vi "Mark Phonation Cutoff.vi"(7 "Error In":errorcluster, 8 "File Path":path, 10 "Pressure/Audio":dynamicdata(graph)) -> (0 "Error Out":errorcluster, 1 "File Path Indicator":path, 2 "Skip?":bool, 3 "Cutoff Pressures":dbl[](array[numeric]))   [LabVIEW 2018, in "AnalysisSupport.lvlib"]
uses:
  AnalysisSupport.lvlib
  <vilib>/Waveform/WDTOps.llb/WDT Get XY Value DBL.vi
panel:
  in  "Jump Button":bool
  in  "Show Audio":bool
  in  "Show EGG":bool
  in  "Undo Button":bool
  out "SPL":dbl
  in  "Help Button":bool
  in  "Add":bool
  out "Interruptions Marked":dbl
  out "Interruption Time":dbl
  in  "Done":bool
  out "Pressure":dbl
  out "EXIT":bool
  out "Enlarged":dynamicdata(graph)
  out "Pressure/Audio":dynamicdata(graph)
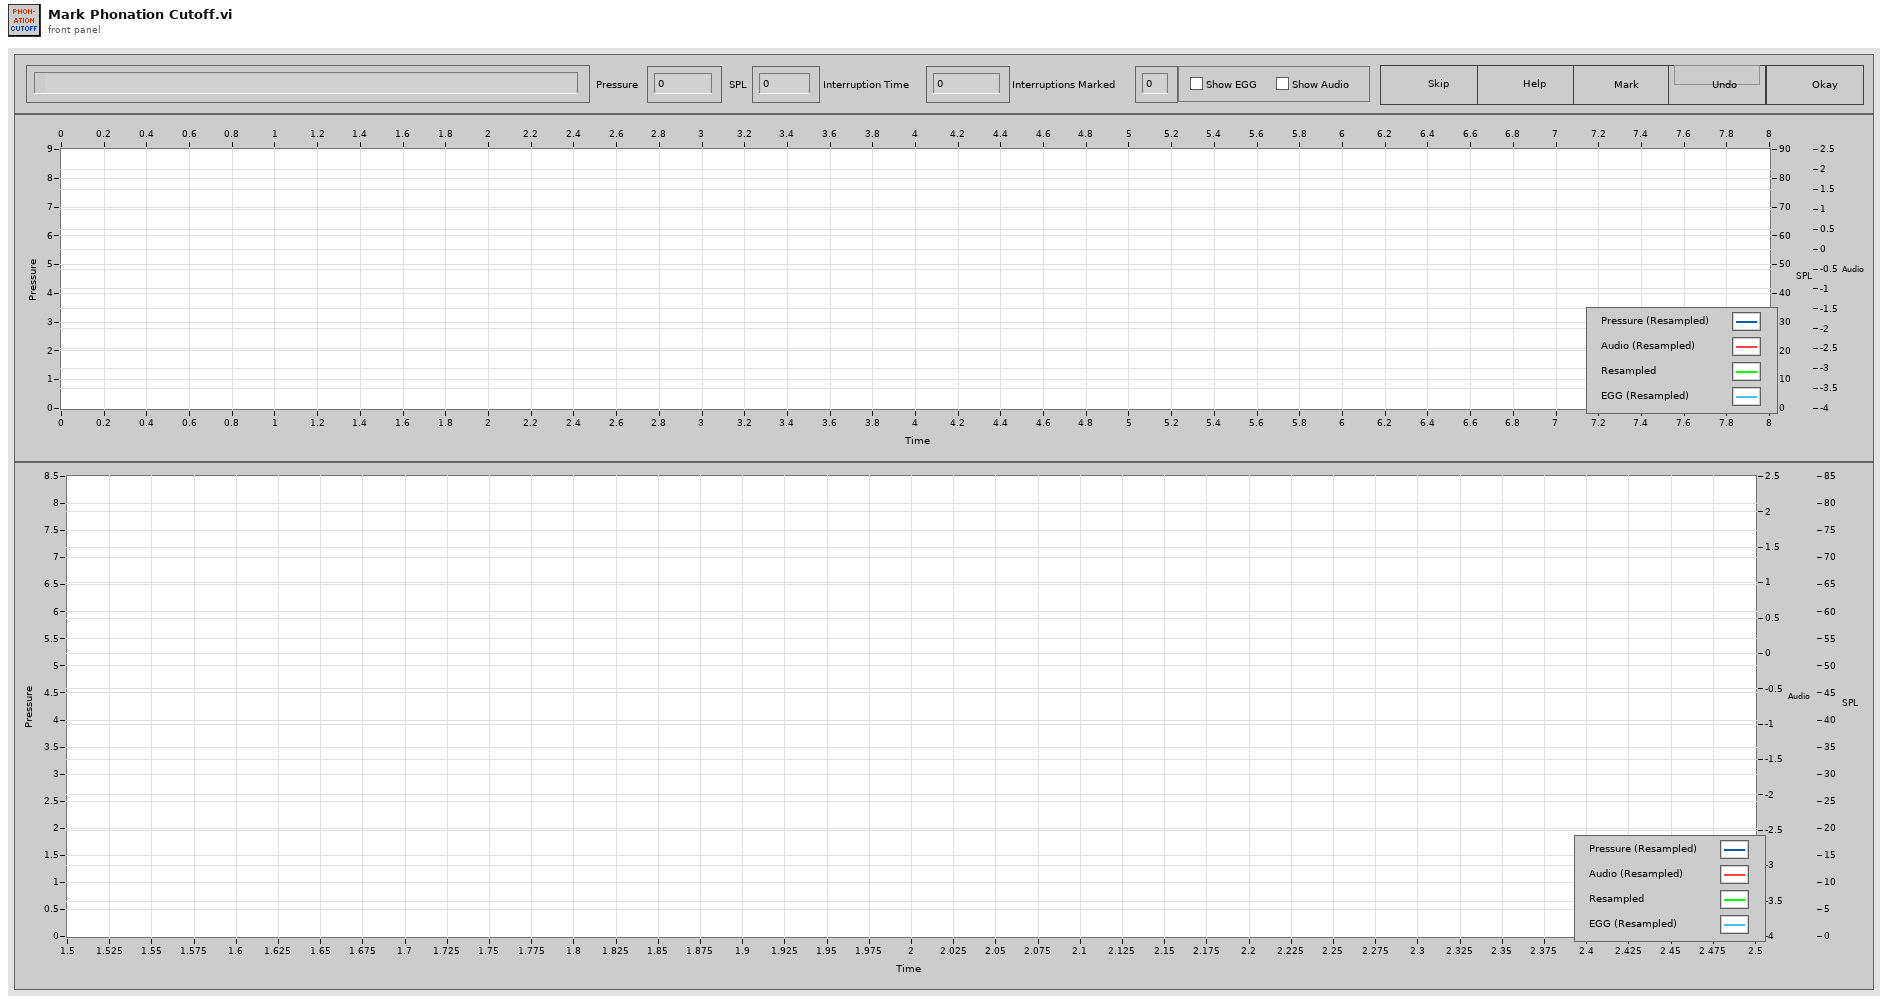
[diagram p1: front panel]
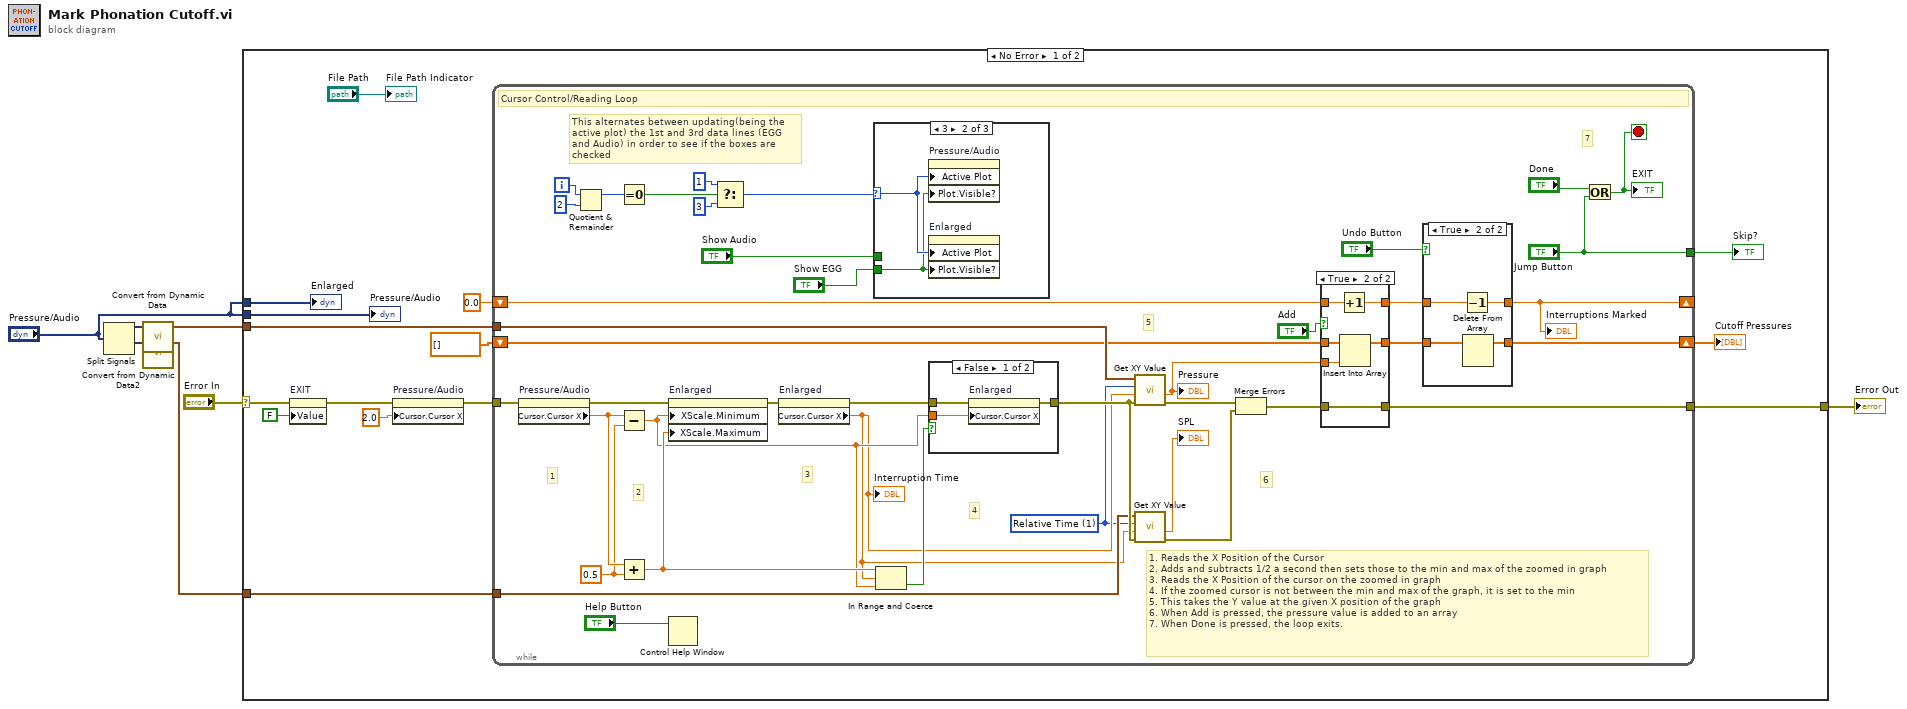
[diagram p0: block diagram]
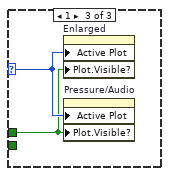
[diagram p3: hidden frame]
diagram:
  n1 = Split Signals("Pressure/Audio") -> (w4:dynamicdata, w2:dynamicdata)  [unwired: 4 in, 2 out]
  n2 = call "Convert from Dynamic Data"("Dynamic Data Type"=w4) -> ("Waveform"=w5:waveform(dbl))  [unwired: 3 in]
  n3 = call "Convert from Dynamic Data2"("Dynamic Data Type"=w2) -> ("Waveform"=w3:waveform(dbl))  [unwired: 3 in]
  n4 = case shown="No Error" "Error In" {
    selector: "Error In" -> [w11 w87]
    tunnel: [w21 w87] -> w7
    tunnel: "Pressure/Audio" -> [w16 _]
    tunnel: "Pressure/Audio" -> [w18 _]
    tunnel: w5 -> [w17 _]
    tunnel: w3 -> [w9 _]
    frame No Error {
      n5 = property on="EXIT" class="Bool (strict)"(error in=w11, "Value"=FALSE ("EXIT")) -> (error out=w10:errorcluster)  [unwired: 1 in, 1 out]
      n6 = property on="Pressure/Audio" class="WFGraph (strict)"(error in=w10, "Cursor.Cursor X"=2.0 ("Cursor.Cursor Position:Cursor X")) -> (error out=w19:errorcluster)  [unwired: 1 in, 1 out]
      n7 = while {
        tunnel: [w53] -> w21
        tunnel: w19 -> [w63]
        tunnel: w17 -> [w62]
        shift-right: [w38] -> _
        shift-left: 0.0 -> [w52]
        shift-right: [w36] -> w13
        shift-left: dbl[] [] ("Cutoff Pressures") -> [w50]
        tunnel: w9 -> [w42]
        tunnel: ["Jump Button"] -> w8
        i -> [w34]
        stop <- w25 stop-if-true
        w40 = u16 1 items=["Samples", "Relative Time"] ("Y position format")
        w59 = 0.5 ("y")
        # "This alternates between updating(being the active plot) the 1st and 3rd data lines (EGG and Audio) in order to see if the boxes are checked"
        # "6"
        # "5"
        # "7"
        # "4"
        # "3"
        # "2"
        # "1"
        # "1. Reads the X Position of the Cursor\n2. Adds and subtracts 1/2 a second then sets those to the min and max of the zoomed in graph\n3. Reads the X Position of the cursor on the zoomed in graph\n4. If the zoomed cursor is not between the min and max of the graph, it is set to the min\n5. This takes the Y value at the given X position of the graph\n6. When Add is pressed, the pressure value is added to an array\n7. When Done is pressed, the loop exits."
        # "Cursor Control/Reading Loop"
        n8 = property on="Pressure/Audio" class="WFGraph (strict)"(error in=w63) -> (error out=w57:errorcluster, "Cursor.Cursor X"=w60:dbl)  [unwired: 1 in, 1 out]
        n9 = Quotient & Remainder(x=w34, y=2) -> (x-y*floor(x/y)=w32:i32)  [unwired: 1 out]
        n10 = Equal To 0?(x=w32) -> (x = 0?=w31:bool)
        n11 = Subtract(x=w60, y=w59) -> (x-y=w54:dbl)
        n12 = Add(x=w60, y=w59) -> (x+y=w58:dbl)
        n13 = Control Help Window(1:"Help Button") -> ()  [unwired: 1 in]
        n14 = property on="Enlarged" class="WFGraph (strict)"(error in=w57, "XScale.Minimum"=w54, "XScale.Maximum"=w58) -> (error out=w56:errorcluster)  [unwired: 1 in, 1 out]
        n15 = Select(t=u32 1 ("Active Plot"), s=w31, f=u32 3 ("Active Plot")) -> (s? t:f=w28:u32)
        n16 = property on="Enlarged" class="WFGraph (strict)"(error in=w56) -> (error out=w55:errorcluster, "Cursor.Cursor X"=w41:dbl)  [unwired: 1 in, 1 out]
        "Interruption Time" <- w41
        n17 = case shown="3" w28 {
          selector: w28 -> [_ w65 w67]
          tunnel: "Show EGG" -> [_ w64 _]
          tunnel: "Show Audio" -> [_ _ w66]
          frame 0, Default {
          }
          frame 3 {
            n18 = property on="Pressure/Audio" class="WFGraph (strict)"("Active Plot"=w65, "Plot.Visible?"=w64) -> ()  [unwired: 2 in, 2 out]
            n19 = property on="Enlarged" class="WFGraph (strict)"("Active Plot"=w65, "Plot.Visible?"=w64) -> ()  [unwired: 2 in, 2 out]
          }
          frame 1 {
            n20 = property on="Enlarged" class="WFGraph (strict)"("Active Plot"=w67, "Plot.Visible?"=w66) -> ()  [unwired: 2 in, 2 out]
            n21 = property on="Pressure/Audio" class="WFGraph (strict)"("Active Plot"=w67, "Plot.Visible?"=w66) -> ()  [unwired: 2 in, 2 out]
          }
        }
        n22 = In Range and Coerce(upper limit=w58, x=w41, lower limit=w54) -> (In Range?=w61:bool)  [unwired: 1 out]
        n23 = case shown="False" w61 {
          tunnel: w55 -> [w76 w77]
          tunnel: [w75 w77] -> w47
          tunnel: w54 -> [w74 _]
          frame False {
            n24 = property on="Enlarged" class="WFGraph (strict)"(error in=w76, "Cursor.Cursor X"=w74) -> (error out=w75:errorcluster)  [unwired: 1 in, 1 out]
          }
          frame True {
          }
        }
        n25 = call-poly <vilib>:"Get XY Value.vi"("error in (no error)"=w47, "Y position"=w41, "Y position format"=w40, "waveform in"=w62) -> ("error out"=w46:errorcluster, "Y value"=w49:dbl)  [unwired: 3 in, 3 out]
        "Pressure" <- w49
        n26 = call-poly <vilib>:"Get XY Value.vi"("error in (no error)"=w47, "Y position"=w41, "Y position format"=w40, "waveform in"=w42) -> ("error out"=w45:errorcluster, "Y value"=→"SPL":dbl)  [unwired: 3 in, 3 out]
        n27 = Merge Errors(w46, w45) -> (w44:errorcluster)
        n28 = case shown="True" "Add" {
          tunnel: w44 -> [w80 w86]
          tunnel: [w80 w86] -> w53
          tunnel: w52 -> [w79 w85]
          tunnel: [w79 w84] -> w39
          tunnel: w50 -> [w78 w83]
          tunnel: w49 -> [_ w82]
          tunnel: [w78 w81] -> w37
          frame False {
          }
          frame True {
            n29 = Increment(x=w85) -> (x+1=w84:dbl)
            n30 = Insert Into Array(array=w83, new element=w82) -> (w81:dbl[])  [unwired: 1 in]
          }
        }
        n31 = case shown="True" "Undo Button" {
          tunnel: w37 -> [w68 w72]
          tunnel: w39 -> [w69 w70]
          tunnel: [w69 w73] -> w38
          tunnel: [w68 w71] -> w36
          frame False {
          }
          frame True {
            n32 = Decrement(x=w70) -> (x-1=w73:dbl)
            n33 = Delete From Array(array=w72) -> (array with subset deleted=w71:dbl[])  [unwired: 2 in, 1 out]
          }
        }
        "Interruptions Marked" <- w38
        n34 = Or(x="Done", y="Jump Button") -> (x .or. y?=w25:bool)
        "EXIT" <- w25
      }
      "Cutoff Pressures" <- w13
      "Skip?" <- w8
      "File Path Indicator" <- "File Path"
      "Enlarged" <- w18
      "Pressure/Audio" <- w16
    }
    frame Error {
    }
  }
  "Error Out" <- w7
